vi "Update DAQ Active.vi"(8 "Error In":errorcluster, 10 "DAQ Active":bool, 11 "LHW-GUI-Actor in":refnum<class "LHW-GUI-Actor.lvclass">) -> (0 "Error Out":errorcluster, 3 "LHW-GUI-Actor out":refnum<class "LHW-GUI-Actor.lvclass">)   [LabVIEW 2014, in "LHW-GUI.lvlib" / "LHW-GUI-Actor.lvclass"]
doc: "Update DAQ Active Status on GUI."
uses:
  LHW-GUI-Actor.lvclass
  LHW-GUI-Actor.lvclass/LHW-GUI-Actor.ctl
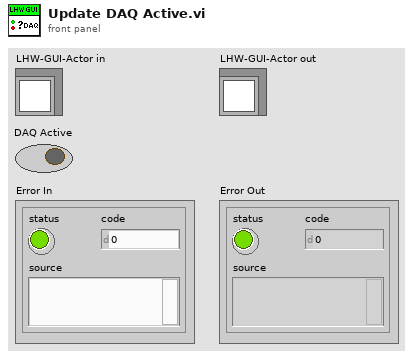
[diagram p1: front panel]
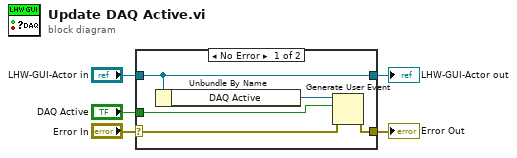
[diagram p0: block diagram]
diagram:
  n1 = case shown="No Error" "Error In" {
    selector: "Error In" -> [w7 w12]
    tunnel: [w6 w12] -> w4
    tunnel: [w10 w11] -> w2
    tunnel: "LHW-GUI-Actor in" -> [w10 w11]
    tunnel: "DAQ Active" -> [w8 _]
    frame No Error {
      n2 = Unbundle By Name(w10) -> ("DAQ Active"=w9:refnum<user-event>)
      n3 = Generate User Event(user event=w9, event data cluster=w8, error in=w7) -> (error out=w6:errorcluster)  [unwired: 1 in, 1 out]
    }
    frame Error {
    }
  }
  "Error Out" <- w4
  "LHW-GUI-Actor out" <- w2
